vi "Serialize Core.vi"(8 "error in":errorcluster, 10 "StrIn":string="{", 11 "variant":variant) -> (0 "error out":errorcluster, 1 "values":string[](array[string]), 2 "StrOut":string, 3 "Variant":variant)   [LabVIEW 2016, in "CVT.lvclass"]
uses:
  CVT.lvclass
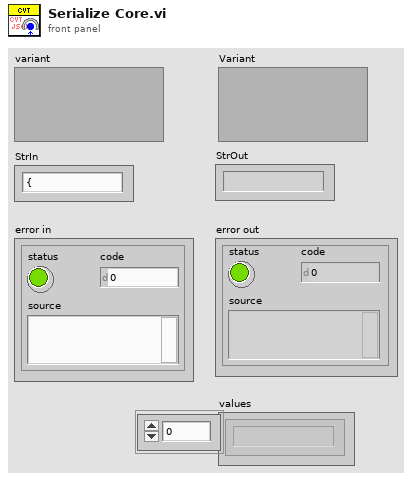
[diagram p1: front panel]
types:
  T1 = typedef "Type Descriptor Enumeration__ogtk.ctl" = enum8{"<Null>", "I8", "I16", "I32", "I64", "U8", "U16", "U32", "U64", "SGL", "DBL", "EXT", "CSG", "CDB", "CXT", "0x0F", "0x10", "0x11", "0x12", "0x13", "0x14", "Enum U8", "Enum U16", "Enum U32", "Enum U64", "SGL PQ", "DBL PQ", "EXT PQ", "CSG PQ", "CDB PQ", "CXT PQ", "0x1F", "0x20", "Boolean", "0x22", "0x23", "0x24", "0x25", "0x26", "0x27", "0x28", "0x29", "0x2A", "0x2B", "0x2C", "0x2D", "0x2E", "0x2F", "String", "0x31", "Path", "Pict", "0x34", "0x35", "0x36", "DAQ", "0x38", "0x39", "0x3A", "0x3B", "0x3C", "0x3D", "0x3E", "0x3F", "Array", "0x41", "0x42", "0x43", "0x44", "0x45", "0x46", "0x47", "0x48", "0x49", "0x4A", "0x4B", "0x4C", "0x4D", "0x4E", "0x4F", "Cluster", "0x51", "0x52", "Variant", "Waveform", "0x55", "0x56", "0x57", "0x58", "0x59", "0x5A", "0x5B", "0x5C", "0x5D", "0x5E", "0x5F", "0x60", "0x61", "0x62", "0x63", "0x64", "0x65", "0x66", "0x67", "0x68", "0x69", "0x6A", "0x6B", "0x6C", "0x6D", "0x6E", "0x6F", "Refnum"}
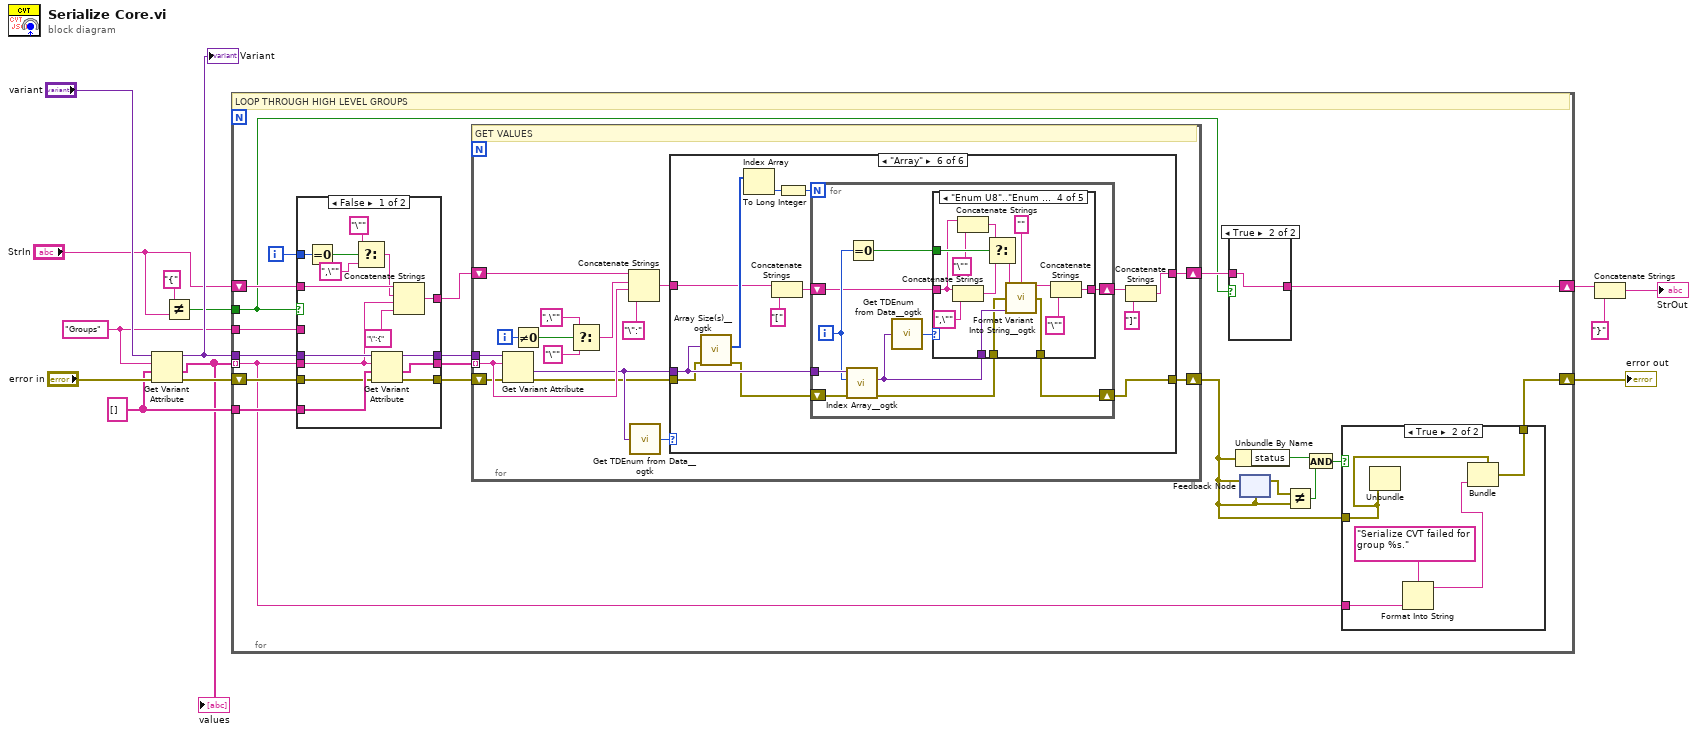
[diagram p0: block diagram]
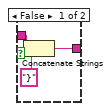
[diagram p3: hidden frame]
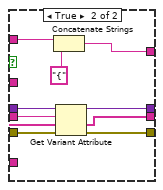
[diagram p4: hidden frame]
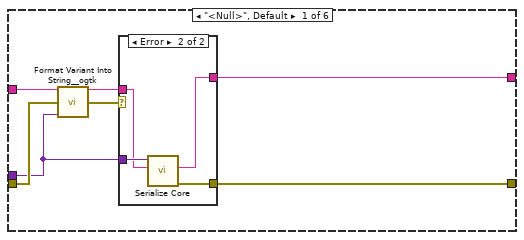
[diagram p5: hidden frame]
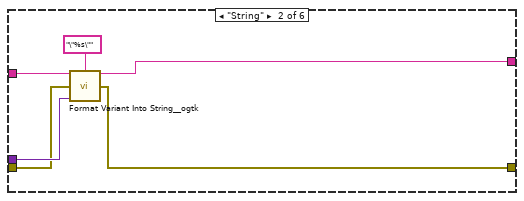
[diagram p7: hidden frame]
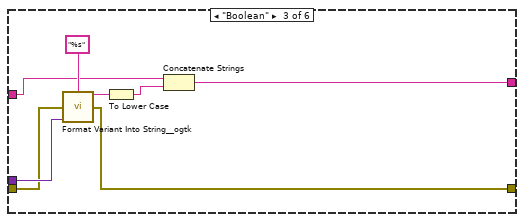
[diagram p8: hidden frame]
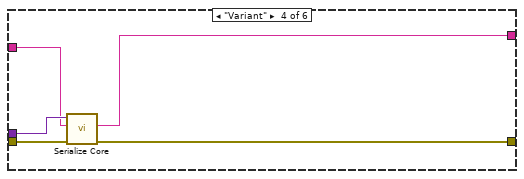
[diagram p9: hidden frame]
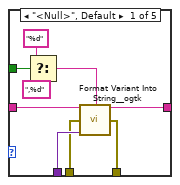
[diagram p11: hidden frame]
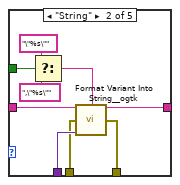
[diagram p12: hidden frame]
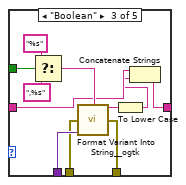
[diagram p13: hidden frame]
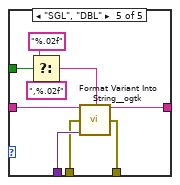
[diagram p14: hidden frame]
diagram:
  w7 = string[] []
  w2 = "Groups" ("name")
  n1 = Get Variant Attribute(Variant="variant", name=w2, default value (empty Variant)=w7, error in="error in") -> (duplicate Variant=w10:variant, value=w6:string[], error out=w13:errorcluster)  [unwired: 1 out]
  "Variant" <- w10
  "values" <- w6
  n2 = Not Equal?(x="{", y="StrIn") -> (x != y?=w1:bool)
  n3 = for {
    tunnel: w10 -> [w34]
    tunnel: w6 -> [w17] mode=indexing
    tunnel: w7 -> [w33]
    shift-right: [w26] -> w8
    shift-left: "StrIn" -> [w30]
    shift-right: [w15] -> w14
    shift-left: w13 -> [w25]
    tunnel: w1 -> [w22]
    tunnel: w2 -> [w23]
    i -> [w28]
    # "LOOP THROUGH HIGH LEVEL GROUPS"
    n4 = case shown="False" w22 {
      tunnel: w34 -> [w59 w69]
      tunnel: w33 -> [w58 w67]
      tunnel: [w57 w64] -> w32
      tunnel: [w56 w68] -> w31
      tunnel: w30 -> [w55 w62]
      tunnel: w17 -> [w54 w63]
      tunnel: [w52 w60] -> w29
      tunnel: w28 -> [w51 _]
      tunnel: w25 -> [w46 w66]
      tunnel: [w45 w65] -> w24
      tunnel: w23 -> [_ _]
      frame False {
        n5 = Equal To 0?(x=w51) -> (x = 0?=w50:bool)
        n6 = Select(t="\"" ("string"), s=w50, f=",\"" ("string")) -> (s? t:f=w47:string)
        n7 = Get Variant Attribute(Variant=w59, name=w54, default value (empty Variant)=w58, error in=w46) -> (duplicate Variant=w56:variant, value=w57:string[], error out=w45:errorcluster)  [unwired: 1 out]
        n8 = Concatenate Strings(w55, w47, w54, "\":{" ("string")) -> (w52:string)
      }
      frame True {
        n9 = Concatenate Strings(w62, "{" ("x")) -> (w60:string)
        n10 = Get Variant Attribute(Variant=w69, name=w63, default value (empty Variant)=w67, error in=w66) -> (duplicate Variant=w68:variant, value=w64:string[], error out=w65:errorcluster)  [unwired: 1 out]
      }
    }
    n11 = for {
      tunnel: w32 -> [w84] mode=indexing
      tunnel: w31 -> [w85]
      shift-right: [w74] -> w27
      shift-left: w29 -> [w82]
      shift-right: [w70] -> w16
      shift-left: w24 -> [w72]
      i -> [w81]
      # "GET VALUES"
      n12 = Get Variant Attribute(Variant=w85, name=w84, error in=w72) -> (value=w75:variant, error out=w71:errorcluster)  [unwired: 1 in, 2 out]
      n13 = Not Equal To 0?(x=w81) -> (x != 0?=w80:bool)
      n14 = Select(t=",\"" ("string"), s=w80, f="\"" ("string")) -> (s? t:f=w77:string)
      n15 = Concatenate Strings(w82, w77, w84, "\":" ("string")) -> (w73:string)
      n16 = call <userlib>:"Get TDEnum from Data__ogtk.vi"("Data"=w75) -> ("Type Descriptor Enumeration"=w76:T1)  [unwired: 4 in]
      n17 = case shown="\"Array\"" w76 {
        tunnel: w75 -> [w88 w104 w112 w117 _ w125]
        tunnel: [w89 w101 w105 w115 w119 w127] -> w74
        tunnel: w73 -> [w92 w102 w106 w113 w119 w131]
        tunnel: w71 -> [w91 w99 w109 w116 w118 w124]
        tunnel: [w86 w100 w110 w114 w118 w122] -> w70
        frame "<Null>", Default {
          n18 = call <userlib>:"Format Variant Into String__ogtk.vi"("Input String"=w92, "error in (no error)"=w91, "Variant"=w88) -> ("Output String"=w90:string, "error out"=w87:errorcluster)  [unwired: 11 in]
          n19 = case shown="Error" w87 {
            selector: w87 -> [w93 _]
            tunnel: w90 -> [w94 w96]
            tunnel: [w94 w95] -> w89
            tunnel: w88 -> [_ w98]
            tunnel: [w93 w97] -> w86
            frame No Error {
            }
            frame Error {
              n20 = call "Serialize Core.vi"("StrIn"=w96, "variant"=w98) -> ("error out"=w97:errorcluster, "StrOut"=w95:string)  [unwired: 6 in, 2 out]
            }
          }
        }
        frame "String" {
          n21 = call <userlib>:"Format Variant Into String__ogtk.vi"("Input String"=w102, "Format String"="\"%s\"", "error in (no error)"=w99, "Variant"=w104) -> ("Output String"=w101:string, "error out"=w100:errorcluster)  [unwired: 10 in]
        }
        frame "Boolean" {
          n22 = call <userlib>:"Format Variant Into String__ogtk.vi"("Format String"="%s", "error in (no error)"=w109, "Variant"=w112) -> ("Output String"=w108:string, "error out"=w110:errorcluster)  [unwired: 11 in]
          n23 = To Lower Case(string=w108) -> (all lower case string=w107:string)
          n24 = Concatenate Strings(w106, w107) -> (w105:string)
        }
        frame "Variant" {
          n25 = call "Serialize Core.vi"("error in"=w116, "StrIn"=w113, "variant"=w117) -> ("error out"=w114:errorcluster, "StrOut"=w115:string)  [unwired: 5 in, 2 out]
        }
        frame "Cluster" {
        }
        frame "Array" {
          n26 = call <userlib>:"Array Size(s)__ogtk.vi"("error in (no error)"=w124, "Array"=w125) -> ("error out"=w123:errorcluster, "Size(s)"=w132:u32[])  [unwired: 7 in, 1 out]
          n27 = Index Array(array=w132) -> (element=w121:u32)  [unwired: 1 in]
          n28 = Concatenate Strings(w131, "[" ("string")) -> (w129:string)
          n29 = To Long Integer(number=w121) -> (32bit integer=w120:i32)
          n30 = for {
            N: w120 -> [_]
            tunnel: w125 -> [w142]
            shift-right: [w136] -> w128
            shift-left: w129 -> [w137]
            shift-right: [w133] -> w122
            shift-left: w123 -> [w138]
            i -> [w141]
            n31 = call <userlib>:"Index Array__ogtk.vi"("error in (no error)"=w138, "Index (1D)"=w141, "MultiD Array"=w142) -> ("error out"=w134:errorcluster, "Array Element"=w135:variant)  [unwired: 7 in]
            n32 = Equal To 0?(x=w141) -> (x = 0?=w140:bool)
            n33 = call <userlib>:"Get TDEnum from Data__ogtk.vi"("Data"=w135) -> ("Type Descriptor Enumeration"=w139:T1)  [unwired: 4 in]
            n34 = case shown="\"Enum U8\"..\"Enum U32\"" w139 {
              tunnel: w140 -> [w149 w158 w169 w185 w194]
              tunnel: w137 -> [w147 w156 w163 w181 w190]
              tunnel: [w145 w154 w161 w175 w188] -> w136
              tunnel: w135 -> [w146 w155 w166 w174 w189]
              tunnel: w134 -> [w144 w153 w165 w173 w187]
              tunnel: [w143 w152 w164 w172 w186] -> w133
              frame "<Null>", Default {
                n35 = Select(t="%d", s=w149, f=",%d") -> (s? t:f=w148:string)
                n36 = call <userlib>:"Format Variant Into String__ogtk.vi"("Input String"=w147, "Format String"=w148, "error in (no error)"=w144, "Variant"=w146) -> ("Output String"=w145:string, "error out"=w143:errorcluster)  [unwired: 10 in]
              }
              frame "String" {
                n37 = Select(t="\"%s\"", s=w158, f=",\"%s\"") -> (s? t:f=w157:string)
                n38 = call <userlib>:"Format Variant Into String__ogtk.vi"("Input String"=w156, "Format String"=w157, "error in (no error)"=w153, "Variant"=w155) -> ("Output String"=w154:string, "error out"=w152:errorcluster)  [unwired: 10 in]
              }
              frame "Boolean" {
                n39 = Select(t="%s", s=w169, f=",%s") -> (s? t:f=w168:string)
                n40 = call <userlib>:"Format Variant Into String__ogtk.vi"("Format String"=w168, "error in (no error)"=w165, "Variant"=w166) -> ("Output String"=w167:string, "error out"=w164:errorcluster)  [unwired: 11 in]
                n41 = To Lower Case(string=w167) -> (all lower case string=w162:string)
                n42 = Concatenate Strings(w163, w162) -> (w161:string)
              }
              frame "Enum U8".."Enum U32" {
                n43 = Concatenate Strings(w181, ",\"" ("string")) -> (w183:string)
                n44 = Concatenate Strings(w181, "\"" ("string")) -> (w182:string)
                n45 = Select(t=w182, s=w185, f=w183) -> (s? t:f=w178:string)
                n46 = call <userlib>:"Format Variant Into String__ogtk.vi"("Input String"=w178, "Format String"="", "error in (no error)"=w173, "Variant"=w174) -> ("Output String"=w176:string, "error out"=w172:errorcluster)  [unwired: 10 in]
                n47 = Concatenate Strings(w176, "\"" ("string")) -> (w175:string)
              }
              frame "SGL", "DBL" {
                n48 = Select(t="%.02f", s=w194, f=",%.02f") -> (s? t:f=w191:string)
                n49 = call <userlib>:"Format Variant Into String__ogtk.vi"("Input String"=w190, "Format String"=w191, "error in (no error)"=w187, "Variant"=w189) -> ("Output String"=w188:string, "error out"=w186:errorcluster)  [unwired: 10 in]
              }
            }
          }
          n50 = Concatenate Strings(w128, "]" ("string")) -> (w127:string)
        }
      }
    }
    n51 = case shown="True" w22 {
      tunnel: w27 -> [w43 w44]
      tunnel: [w41 w44] -> w26
      frame False {
        n52 = Concatenate Strings(w43, "}" ("string")) -> (w41:string)
      }
      frame True {
      }
    }
    n53 = Unbundle By Name(w16) -> ("status"=w19:bool)
    n54 = feedback-in #1(w16) -> ()
    n55 = feedback #1(w16) -> (w21:errorcluster)
    n56 = Not Equal?(x=w21, y=w16) -> (x != y?=w20:bool)
    n57 = And(x=w19, y=w20) -> (x .and. y?=w18:bool)
    n58 = case shown="True" w18 {
      tunnel: w16 -> [w35 w38]
      tunnel: w17 -> [_ w40]
      tunnel: [w35 w36] -> w15
      frame False {
      }
      frame True {
        n59 = Unbundle(w38) -> ()  [unwired: 3 out]
        n60 = Format Into String(format string="Serialize CVT failed for group %s.", w40) -> (resulting string=w37:string)  [unwired: 2 in, 1 out]
        n61 = Bundle(cluster=w38, "source"=w37) -> (w36:errorcluster)  [unwired: 2 in]
      }
    }
  }
  "error out" <- w14
  n62 = Concatenate Strings(w8, "}" ("string")) -> (→"StrOut":string)
